vi "available tags menu.vi"(4 "Coords":T9, 5 "parent vi reference":refnum<vi>, 6 "Screen":bool, 8 "error in":errorcluster, 9 "channel to map to":refnum<class "TBM channel.lvclass">, 10 "object ref":T1, 11 "references in":T2) -> (0 "error out":errorcluster, 3 "references out":T2)   [LabVIEW 2013, in "tag select module editor node.lvclass"]
uses:
  tag select module editor node.lvclass
  <vilib>/NI/Tag Bus Module Framework/channel/TBM channel.lvclass
  <vilib>/Utility/miscctls.llb/LVPoint32TypeDef.ctl
  references.ctl
  <vilib>/NI/Configuration Framework/Node/StopEvent.ctl
  <vilib>/NI/Configuration Framework/Node/RefreshUIEvent.ctl
  <vilib>/NI/Configuration Framework/Node/CacheState.ctl
  <vilib>/NI/Configuration Framework/Node/NodeChangeEvent.ctl
  <vilib>/NI/Configuration Framework/Node/NodeRef.ctl
  <vilib>/NI/Configuration Framework/Node/NISE_CEF_Node.lvclass
  <vilib>/NI/Tag Bus Data Framework/control module/editor node/channel action event.ctl
  <vilib>/NI/Tag Bus Data Framework/control module/editor node/dialog output action.ctl
  <vilib>/NI/Tag Bus/tag/tag descriptor.lvclass
  <vilib>/NI/AMC/Message Queue.ctl
  <vilib>/NI/AMC/Message.ctl
  <vilib>/NI/Tools/Keyed Array/KeyedArray.ctl
  <vilib>/NI/Configuration Framework/Node/UserEventRef.ctl
  <vilib>/NI/Configuration Framework/Controls/EventCluster.ctl
  object ref.ctl
  <vilib>/NI/Tag Bus Data Framework/Configuration Editor/Classes/Engine Parent/Engine Parent Editor Node.lvclass
  <vilib>/NI/Tag Bus Data Framework/Configuration Editor/Classes/Engine Parent/read engine configuration.vi
  <vilib>/NI/Module Execution Interface/Engine Configuration/engine configuration.lvclass
  <vilib>/NI/Tag Bus Data Framework/control module/editor node/control module editor.lvclass
  <vilib>/NI/Tools/Keyed Array/Tools_KeyedArray.lvlib
  <vilib>/NI/AMC/AMC.lvlib
  <vilib>/NI/Configuration Framework/NISE_CEF_TreeControl.lvlib
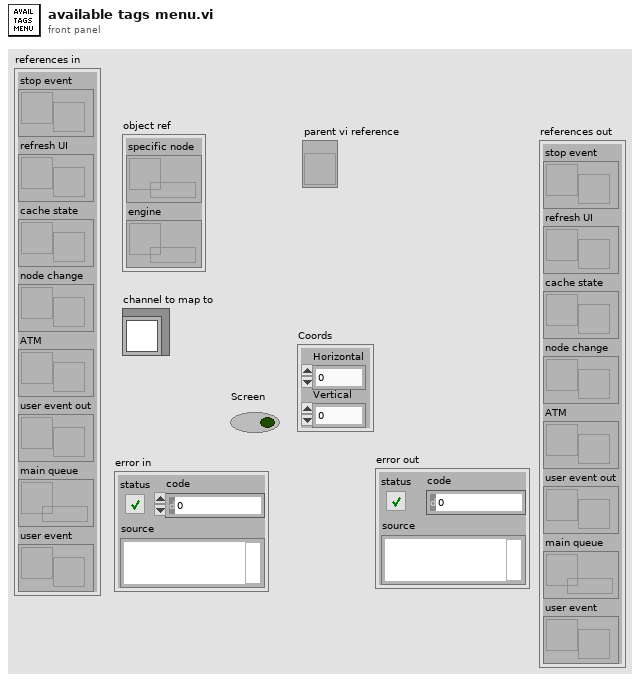
[diagram p1: front panel]
types:
  T1 = typedef "tag select module editor node.lvclass/object ref.ctl" = cluster{"specific node":refnum<data-value>, "engine":refnum<data-value>}
  T2 = typedef "tag select module editor node.lvclass/references.ctl" = cluster{"stop event":T3, "refresh UI":T4, "cache state":T5, "node change":T6, "ATM":refnum<user-event>, "user event out":refnum<user-event>, "main queue":T7, "user event":T8}
  T3 = typedef "NISE_CEF_Node.lvclass/StopEvent.ctl" = refnum<user-event>
  T4 = typedef "NISE_CEF_Node.lvclass/RefreshUIEvent.ctl" = refnum<user-event>
  T5 = typedef "NISE_CEF_Node.lvclass/CacheState.ctl" = refnum<user-event>
  T6 = typedef "NISE_CEF_Node.lvclass/NodeChangeEvent.ctl" = refnum<user-event>
  T7 = typedef "AMC.lvlib/Message Queue.ctl" = refnum<queue>
  T8 = typedef "NISE_CEF_Node.lvclass/UserEventRef.ctl" = refnum<user-event>
  T9 = typedef "LVPoint32TypeDef.ctl" = cluster{"Horizontal":i32, "Vertical":i32}
  T10 = enum32{"Invalid", "Standard", "Closed", "Hidden", "Minimized", "Maximized"}
  T11 = typedef "LVRectTypeDef.ctl" = cluster{"Left":i16, "Top":i16, "Right":i16, "Bottom":i16}
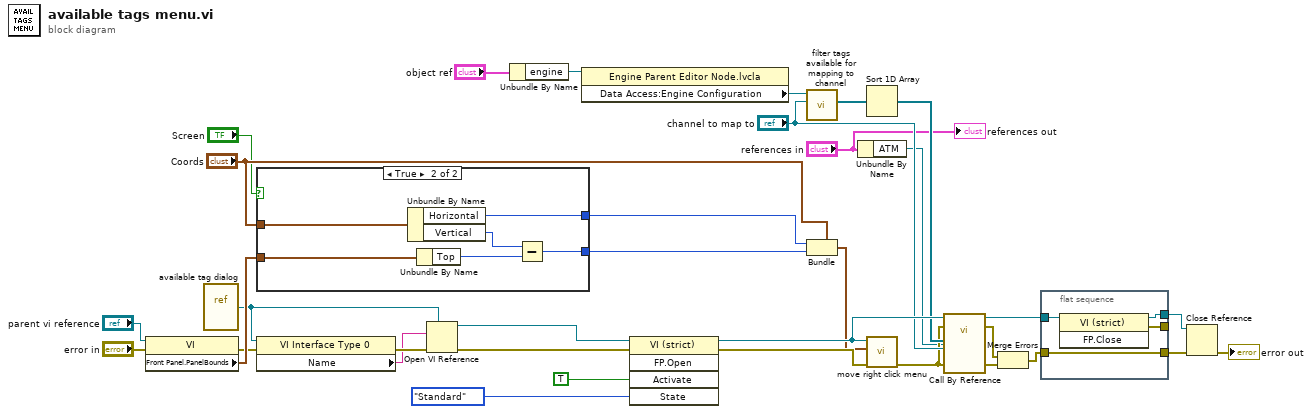
[diagram p0: block diagram]
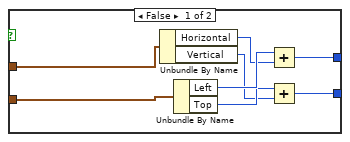
[diagram p2: hidden frame]
diagram:
  n1 = property class="VI"(reference="parent vi reference", error in="error in") -> (error out=w14:errorcluster, "Front Panel.PanelBounds"=w33:T11)  [unwired: 1 out]
  n2 = vi-ref "available tag dialog.vi"() -> (w21:refnum<vi>)
  n3 = case shown="True" "Screen" {
    tunnel: w33 -> [w42 w46]
    tunnel: [w39 w47] -> w32
    tunnel: [w36 w43] -> w31
    tunnel: "Coords" -> [w35 w48]
    frame False {
      n4 = Unbundle By Name(w35) -> ("Horizontal"=w40:i32, "Vertical"=w37:i32)
      n5 = Unbundle By Name(w42) -> ("Left"=w41:i16, "Top"=w38:i16)
      n6 = Add(x=w41, y=w40) -> (x+y=w39:i32)
      n7 = Add(x=w38, y=w37) -> (x+y=w36:i32)
    }
    frame True {
      n8 = Unbundle By Name(w48) -> ("Horizontal"=w47:i32, "Vertical"=w45:i32)
      n9 = Unbundle By Name(w46) -> ("Top"=w44:i16)
      n10 = Subtract(x=w45, y=w44) -> (x-y=w43:i32)
    }
  }
  n11 = property class="VI Interface Type 0"(reference=w21, error in=w14) -> (error out=w28:errorcluster, "Name"=w27:string)  [unwired: 1 out]
  n12 = Open VI Reference(type specifier VI Refnum (for type only)=w21, vi path=w27, error in (no error)=w28) -> (vi reference=w25:refnum<vi>, error out=w26:errorcluster)  [unwired: 3 in]
  n13 = Unbundle By Name("object ref") -> ("engine"=w2:refnum<data-value>)
  n14 = property class="Engine Parent Editor Node.lvcla"(reference=w2) -> ("Data Access:Engine Configuration"=w4:refnum<class "engine configuration.lvclass">)  [unwired: 1 in, 2 out]
  n15 = invoke class="VI (strict)" method="FP.Open"(reference=w25, error in=w26, "Activate"=TRUE ("Activate?"), "State"=T10."Standard") -> (reference out=w20:refnum<vi>, error out=w22:errorcluster)  [unwired: 1 in, 3 out]
  n16 = call <vilib>:"filter tags available for mapping to channel.vi"("channel to map to"="channel to map to", "engine configuration in"=w4) -> ("filtered tags"=w34:refnum<class "tag descriptor.lvclass">[])  [unwired: 8 in, 1 out]
  n17 = Bundle(cluster="Coords", "Horizontal"=w32, "Vertical"=w31) -> (w11:T9)
  n18 = Unbundle By Name("references in") -> ("ATM"=w5:refnum<user-event>)
  n19 = Sort 1D Array(array=w34) -> (sorted array=w12:refnum<class "tag descriptor.lvclass">[])
  n20 = call <vilib>:"move right click menu.vi"("error in"=w22, "Point32"=w11, "VI"=w20) -> ("error out"=w8:errorcluster)  [unwired: 8 in]
  n21 = call-by-ref "?"(reference=w20, error in=w8, "channel action event"=w5, "error in"=w8, "channel to map to"="channel to map to", "filtered tags"=w12) -> (reference out=w18:refnum<vi>, error out=w19:errorcluster, 0:"error out"=w7:errorcluster)  [unwired: 7 in]
  n22 = Merge Errors(w19, w7) -> (w10:errorcluster)
  n23 = flat-sequence {
    tunnel: w18 -> [w52]
    tunnel: [w51] -> w17
    tunnel: [w50] -> _
    tunnel: w10 -> [w49]
    tunnel: [w49] -> w9
    frame #0 {
      n24 = invoke class="VI (strict)" method="FP.Close"(reference=w52) -> (reference out=w51:refnum<vi>, error out=w50:errorcluster)  [unwired: 2 in, 1 out]
    }
  }
  n25 = Close Reference(reference=w17, error in (no error)=w9) -> (error out=→"error out":errorcluster)
  "references out" <- "references in"
